vi "Analog Input.vi"() -> ()   [LabVIEW 2019]
doc: "Analog Input Example\n\nThis example will read voltages from an analog channel and display it on a chart. It will also display the average voltage over time. \n\nThe values for Average Bits and Samples Per Second on the front panel can be set while the VI is running.\n\nThis example expects a USB cable connected from your development PC to the Type B USB Jack (next to the power input) on the roboRIO."
uses:
  <vilib>/Rock Robotics/SystemInterfaces/AI/FPGA_AIChannel.ctl
panel:
  in  "Samples Per Second":dbl=1000.0
  in  "Average Bits":u8=3 max=15
  in  "Channel":T1=enum."AI 1"
  out "Voltage Display":cluster{"Value":dbl, "Voltage":dbl}(graph)
  out "Average Voltage":dbl
  out "Voltage":dbl
  in  "stop":bool
  # "Set this input before running."
  # "These can be set while running."
  # "This chart displays the voltage and average voltage over time."
  # "This shows wiring for a typical analog input using a potentiometer.  In this case the potentiometer is being powered with 5 volts, and the Signal returned will vary from 0 to 5 volts"
  # "potentiometer"
  # "Gnd"
  # "S"
  # "V"
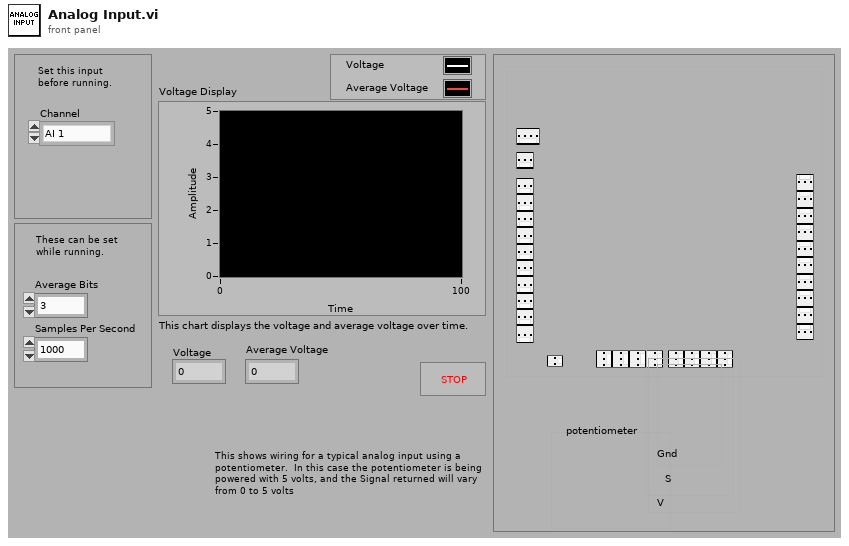
[diagram p1: front panel]
types:
  T1 = typedef "FPGA_AIChannel.ctl" = enum8{"AI 0", "AI 1", "AI 2", "AI 3", "AI MXP 0", "AI MXP 1", "AI MXP 2", "AI MXP 3", "Invalid"}
  T2 = typedef "WPI_AnalogChannelDevRef.ctl" = cluster{"DevStatus":errorcluster, "Analog Channel":T1}
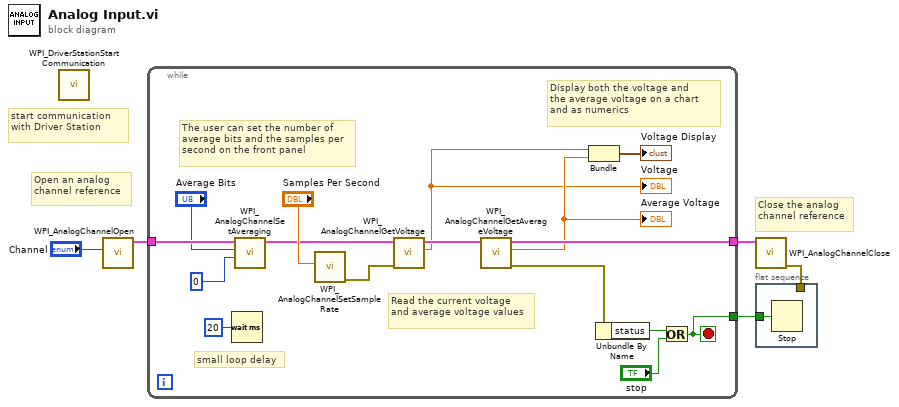
[diagram p0: block diagram]
diagram:
  # "start communication with Driver Station"
  # "Close the analog\nchannel reference"
  # "Open an analog channel reference"
  n1 = call <vilib>:"WPI_DriverStationStart Communication.vi"() -> ()  [unwired: 3 in, 9 out]
  n2 = call <vilib>:"WPI_AnalogChannelOpen.vi"("Analog Channel"="Channel") -> ("AIDeviceRef"=w5:T2)  [unwired: 2 in, 8 out]
  n3 = while {
    tunnel: w5 -> [w15]
    tunnel: [w20] -> w4
    tunnel: [w6] -> w2
    stop <- w6 stop-if-true
    # "small loop delay"
    # "Read the current voltage\nand average voltage values"
    # "Display both the voltage and\nthe average voltage on a chart\nand as numerics"
    # "The user can set the number of \naverage bits and the samples per\nsecond on the front panel"
    n4 = Wait (ms)(milliseconds to wait=u32 20) -> ()  [unwired: 1 out]
    n5 = call <vilib>:"WPI_AnalogChannelSetAveraging.vi"("OversampleBits"=u8 0, "AverageBits"="Average Bits", "AIDeviceRef"=w15) -> ("AIDeviceRef"=w9:T2)  [unwired: 1 in, 7 out]
    n6 = call <vilib>:"WPI_AnalogChannelSetSampleRate.vi"("Samples Per Second (per channel)"="Samples Per Second") -> ("error out"=w7:errorcluster)  [unwired: 4 in, 6 out]
    n7 = call <vilib>:"WPI_AnalogChannelGetVoltage.vi"("error in (no error)"=w7, "AIDeviceRef"=w9) -> ("Voltage"=w18:dbl, "AIDeviceRef"=w21:T2)  [unwired: 8 out]
    "Voltage" <- w18
    n8 = call <vilib>:"WPI_AnalogChannelGetAverageVoltage.vi"("AIDeviceRef"=w21) -> ("error out"=w8:errorcluster, "Voltage"=w19:dbl, "AIDeviceRef"=w20:T2)  [unwired: 1 in, 7 out]
    "Average Voltage" <- w19
    n9 = Bundle("Voltage"=w18, "Voltage"=w19) -> (→"Voltage Display":cluster{"Voltage":dbl, "Voltage":dbl})  [unwired: 1 out]
    n10 = Unbundle By Name(w8) -> ("status"=w13:bool)
    n11 = Or(x=w13, y="stop") -> (x .or. y?=w6:bool)
  }
  n12 = call <vilib>:"WPI_AnalogChannelClose.vi"("AIDeviceRef"=w4) -> ("error out"=w1:errorcluster)  [unwired: 1 in, 9 out]
  n13 = flat-sequence {
    tunnel: w2 -> [w22]
    tunnel: w1 -> [_]
    frame #0 {
      n14 = Stop(stop? (T)=w22) -> ()
    }
  }
